vi "Queue Data to Array.vi"(11 "elements":cluster{"register values":dbl[][]}[](array[cluster])) -> (3 "Array":dbl[][](array[numeric]))   [LabVIEW 2020]
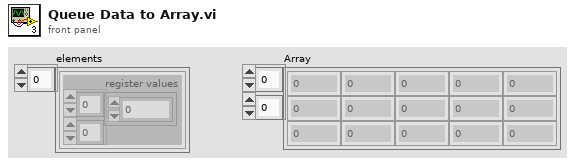
[diagram p1: front panel]
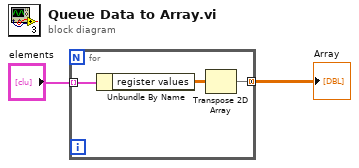
[diagram p0: block diagram]
diagram:
  n1 = for {
    tunnel: "elements" -> [w5] mode=indexing
    tunnel: [w3] -> w2 mode=concatenating
    n2 = Unbundle By Name(w5) -> ("register values"=w4:dbl[][])
    n3 = Transpose 2D Array(2D array=w4) -> (transposed array=w3:dbl[][])
  }
  "Array" <- w2
